vi "Write Analysis Params.vi"(8 "error in (no error)":errorcluster, 10 "Analysis Params":T1, 11 "Optical Spectrum Analyzer in":refnum<class "Optical Spectrum Analyzer.lvclass">) -> (0 "error out":errorcluster, 3 "Optical Spectrum Analyzer out":refnum<class "Optical Spectrum Analyzer.lvclass">)   [LabVIEW 2018, in "Optical Spectrum Analyzer.lvlib" / "Optical Spectrum Analyzer.lvclass"]
uses:
  Optical Spectrum Analyzer.lvclass
  Optical Spectrum Analyzer.lvclass/Optical Spectrum Analyzer.ctl
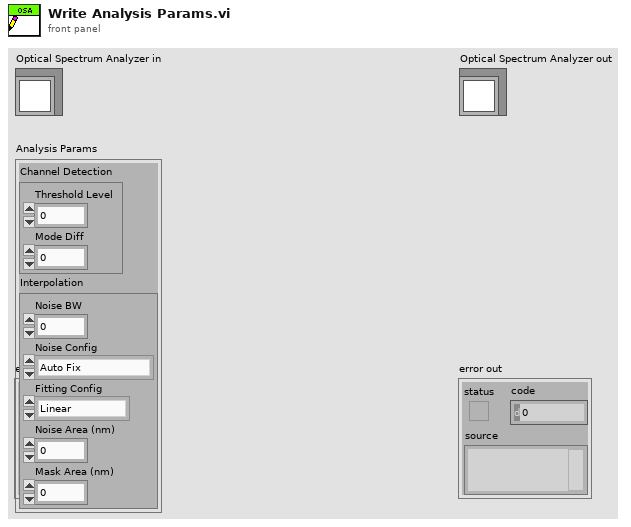
[diagram p1: front panel]
types:
  T1 = cluster{"Channel Detection":cluster{"Threshold Level":dbl, "Mode Diff":dbl}, "Interpolation":cluster{"Noise BW":dbl, "Noise Config":enum16{"Auto Fix", "Manual Fix", "Auto Center", "Manual Center"}, "Fitting Config":enum16{"Linear", "Gauss", "Lorenz", "3rd Poly", "4th Poly", "5th Poly"}, "Noise Area (nm)":dbl, "Mask Area (nm)":dbl}}
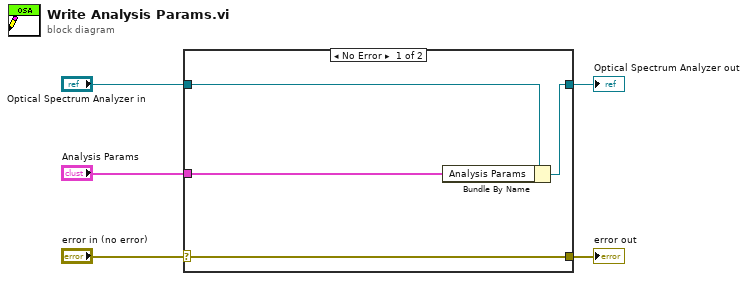
[diagram p0: block diagram]
diagram:
  n1 = case shown="No Error" "error in (no error)" {
    selector: "error in (no error)" -> [w9 w10]
    tunnel: [w9 w10] -> w4
    tunnel: [w7 w11] -> w2
    tunnel: "Optical Spectrum Analyzer in" -> [w8 w11]
    tunnel: "Analysis Params" -> [w6 _]
    frame No Error {
      n2 = Bundle By Name(cluster=w8, "Analysis Params"=w6) -> (w7:refnum<class "Optical Spectrum Analyzer.lvclass">)
    }
    frame Error {
    }
  }
  "error out" <- w4
  "Optical Spectrum Analyzer out" <- w2
